vi "test_Set and Get 9225.vi"(8 "error in (no error)":errorcluster, 11 "TestCase in":refnum<class "Scan Engine Scripting API Custom Device Unit Tests.lvclass">) -> (0 "error out":errorcluster, 3 "TestCase out":refnum<class "Scan Engine Scripting API Custom Device Unit Tests.lvclass">)   [LabVIEW 2020, in "Scan Engine Scripting API Custom Device Unit Tests.lvclass"]
uses:
  Scan Engine Scripting API Custom Device Unit Tests.lvclass
  Scripting/Modules/NI 9225/NI 9225.lvclass
  C:/Users/nitest/Desktop/Git 2020/niveristand-scan-engine-ethercat-custom-device/Custom Device Source/Scripting/Modules/Module/Module.lvclass
  Scan Engine Scripting API Custom Device Unit Tests.lvclass/Scan Engine Scripting API Custom Device Unit Tests.ctl
  83415135-542a-4f08-98f1-586d031c4d33.vi
  Shared/Utility/Set Error.vi
  <vilib>/Utility/error.llb/Clear Errors.vi
  Scripting/Utility/Convert Slot Configuration to 9212.vi
  Scripting/Utility/Convert Slot Configuration to 9213.vi
  Includes/Modules.lvlibp/SD Module/SD Module.lvclass
  C:/Users/nitest/Desktop/Git 2020/niveristand-scan-engine-ethercat-custom-device/Includes/Modules.lvlibp/RSI Module/RSI Module.lvclass
  Scripting/Modules/NI 9212/NI 9212.lvclass
  Scripting/Modules/NI 9213/NI 9213.lvclass
  Scripting/Modules/NI 9224/NI 9224.lvclass
  Scripting/Modules/NI 9228/NI 9228.lvclass
  Includes/Modules.lvlibp/RSI Module/Read Module Page Property.vi
  Includes/Modules.lvlibp/RSI Module/Read Model.vi
  Scripting/Utility/Convert Module Model to Module Class.vi
  Includes/Modules.lvlibp/SD Module/Read DIO mode.vi
  Includes/Modules.lvlibp/RSI Module/Read Channels.vi
  Scripting/Utility/Convert to DI Module.vi
  Scripting/Utility/Convert to DO Module.vi
  Scripting/Utility/Convert to CI PWM Module.vi
  Scripting/Utility/Convert to CDO Module.vi
  Scripting/Utility/Convert to PWM Module.vi
  Shared/Globals/Error Strings.vi
  Scripting/Utility/Get Channel Names and Default Values for Slot.vi
  Scripting/Modules/NI 9212/Create NI 9212.vi
  Scripting/Modules/NI 9213/Create NI 9213.vi
  Scripting/Utility/Convert to AI Module.vi
  Scripting/Utility/Convert to AI Vrms Module.vi
  Scripting/Utility/Convert to AI Arms Module.vi
  Scripting/Utility/Convert to DIO Module.vi
  Scripting/Modules/Module/Module.lvclass
  Includes/Modules.lvlibp/9212/9212.lvclass
  Includes/Modules.lvlibp/9213/9213.lvclass
  Includes/Modules.lvlibp/9224/9224.lvclass
  <vilib>/addons/_JKI Toolkits/VI Tester/TestCase.llb/TestCase.lvclass
  Scripting/Scan Engine Scripting.lvlib
  C:/Program Files (x86)/National Instruments/LabVIEW 2020/vi.lib/addons/_JKI Toolkits/VI Tester/TestCase.llb/TestCase.lvclass
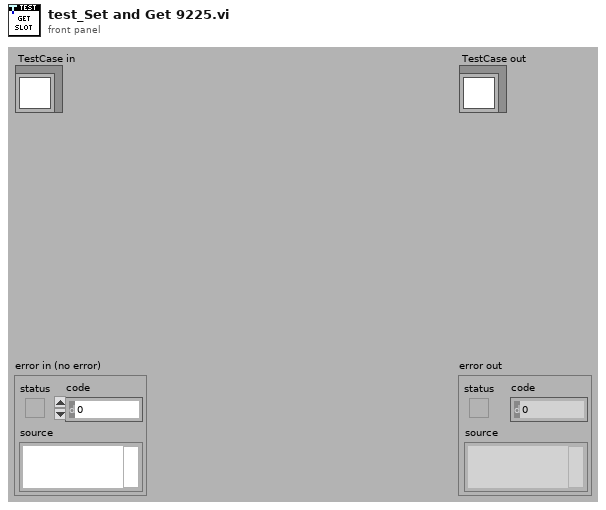
[diagram p1: front panel]
types:
  T1 = typedef "Custom Device API.lvlib/Custom Device Item Ref.ctl" = u64
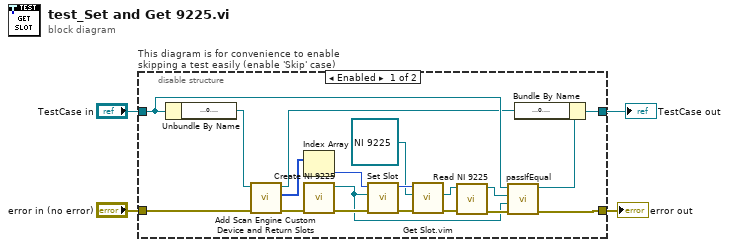
[diagram p0: block diagram]
diagram:
  n1 = disable-structure "This diagram is for convenience to enable skipping a test easily (enable 'Skip' case)" shown="Enabled" {
    disable-tunnel: "TestCase in" -> [w17 w27]
    disable-tunnel: [w19 w25] -> w1
    disable-tunnel: [w13 w26] -> w3
    disable-tunnel: "error in (no error)" -> [w23 w24]
    frame Enabled {
      n2 = Unbundle By Name(w17) -> ("target ref"=w22:refnum<k24>)
      n3 = call "Add Scan Engine Custom Device and Return Slots.vi"("error in"=w23, "target ref in"=w22) -> ("error out"=w15:errorcluster, "slot refs"=w21:T1[], "target ref out"=w16:refnum<k24>)  [unwired: 7 in]
      n4 = Index Array(array=w21) -> (element=w20:T1)  [unwired: 1 in]
      n5 = call "Create NI 9225.vi"("error in"=w15) -> ("error out"=w14:errorcluster, "NI 9225 out"=w8:refnum<class "NI 9225.lvclass">)  [unwired: 9 in]
      n6 = call "Set Slot.vi"("error in"=w14, "module"=w8, "slot ref in"=w20) -> ("error out"=w18:errorcluster, "slot ref out"=w9:T1)  [unwired: 7 in]
      n7 = call "Get Slot.vim"("error in"=w18, "module type"=refnum<class "NI 9225.lvclass"> refnum ("NI 9225 out"), "slot ref in"=w9) -> ("error out"=w6:errorcluster, "module"=w7:refnum<class "NI 9225.lvclass">)  [unwired: 5 in, 2 out]
      n8 = call "Read NI 9225.vi"("error in"=w6, "NI 9225 in"=w7) -> ("error out"=w11:errorcluster, "NI 9225 out"=w12:refnum<class "NI 9225.lvclass">)  [unwired: 7 in, 1 out]
      n9 = call-dynamic "passIfEqual.vi"("error in (no error)"=w11, "y"=w8, "x"=w12, "TestCase in"=w17) -> ("error out"=w13:errorcluster, "TestCase out"=w10:refnum<class "Scan Engine Scripting API Custom Device Unit Tests.lvclass">)  [unwired: 6 in]
      n10 = Bundle By Name(cluster=w10, "target ref"=w16) -> (w19:refnum<class "Scan Engine Scripting API Custom Device Unit Tests.lvclass">)
    }
    frame Disabled {
      # "skip test result while test is under development"
      n11 = call <vilib>:"skip.vi"("error in (no error)"=w24, "TestCase in"=w27) -> ("error out"=w26:errorcluster, "TestCase out"=w25:refnum<class "Scan Engine Scripting API Custom Device Unit Tests.lvclass">)  [unwired: 8 in]
    }
  }
  "error out" <- w3
  "TestCase out" <- w1
